vi "StimCompOKN.vi"(8 "Offset":dbl format="%#_13g", 9 "Amp":dbl=10.0 format="%#_13g", 10 "frequency":dbl=0.25 format="%#_13g", 11 "sampling info":cluster{"Fs":dbl, "#s":dbl}={"Fs"=100.0, "#s"=400.0}) -> (0 "ComplexStim":T1, 3 "Stim":dbl[][](array[numeric]))   [LabVIEW 2016]
uses:
  <vilib>/measure/NI_MABase.lvlib
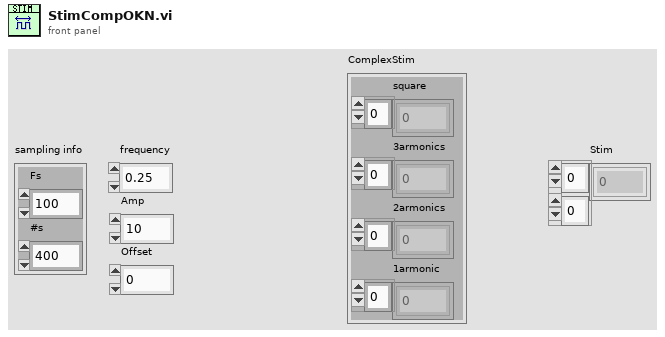
[diagram p1: front panel]
types:
  T1 = cluster{"square":dbl[], "3armonics":dbl[], "2armonics":dbl[], "1armonic":dbl[]}
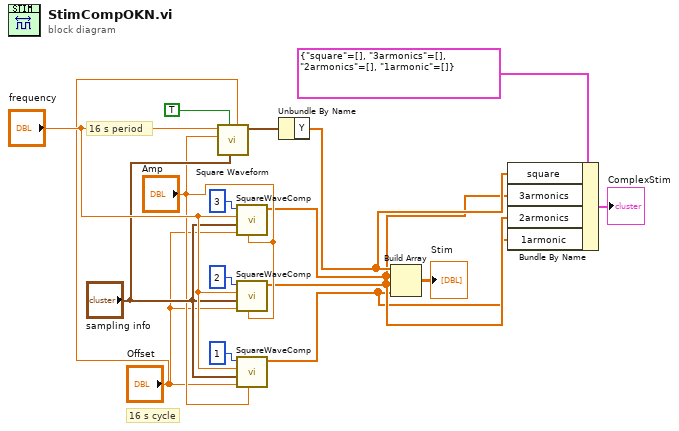
[diagram p0: block diagram]
diagram:
  # "16 s period"
  # "16 s cycle"
  n1 = call <vilib>:"Square Waveform.vi"("offset"="Offset", "sampling info"="sampling info", "reset signal"=TRUE, "amplitude"="Amp", "frequency"="frequency") -> ("signal out"=w16:waveform(dbl))  [unwired: 5 in, 1 out]
  n2 = call "SquareWaveComp.vi"("Amp"="Amp", "Offset"="Offset", "sampling info"="sampling info", "frequency"="frequency", "Components"=3) -> ("Decomposed"=w4:dbl[])  [unwired: 6 in]
  n3 = call "SquareWaveComp.vi"("Amp"="Amp", "Offset"="Offset", "sampling info"="sampling info", "frequency"="frequency", "Components"=2) -> ("Decomposed"=w3:dbl[])  [unwired: 6 in]
  n4 = call "SquareWaveComp.vi"("Amp"="Amp", "Offset"="Offset", "sampling info"="sampling info", "frequency"="frequency", "Components"=1) -> ("Decomposed"=w2:dbl[])  [unwired: 6 in]
  n5 = Unbundle By Name(w16) -> ("Y"=w5:dbl[])
  n6 = Build Array(w5, w4, w3, w2) -> (→"Stim":dbl[][])
  n7 = Bundle By Name(cluster=T1 {"square"=[], "3armonics"=[], "2armonics"=[], "1armonic"=[]}, "square"=w5, "3armonics"=w4, "2armonics"=w3, "1armonic"=w2) -> (→"ComplexStim":T1)
